vi "getServerCapability.vi"(8 "error in (no error)":errorcluster, 10 "ProtocolId in":string, 11 "IDeviceInfo in":refnum<class "IDeviceInfo.lvclass">) -> (0 "error out":errorcluster, 1 "ServerCapability out":refnum<class "IServerCapability.lvclass">, 2 "ProtocolId out":string, 3 "IDeviceInfo out":refnum<class "IDeviceInfo.lvclass">)   [LabVIEW 2022 SP3, in "openDAQ.lvlib" / "IBaseObject.lvlib" / "IPropertyObject.lvlib" / "IDeviceInfo.lvlib" / "IDeviceInfo.lvclass"]
uses:
  <instrlib>/openDAQ/Public/Classes/IDeviceInfo/IDeviceInfo.lvclass
  <instrlib>/openDAQ/Public/Classes/IDeviceInfo/IDeviceInfo.lvclass/IDeviceInfo.ctl
  <instrlib>/openDAQ/Public/Classes/daqCoreTypes/IString/IString.lvclass
  <instrlib>/openDAQ/Public/Classes/IServerCapability/IServerCapability.lvclass
  <instrlib>/openDAQ/Binaries/Windows/x86/copendaq32.dll
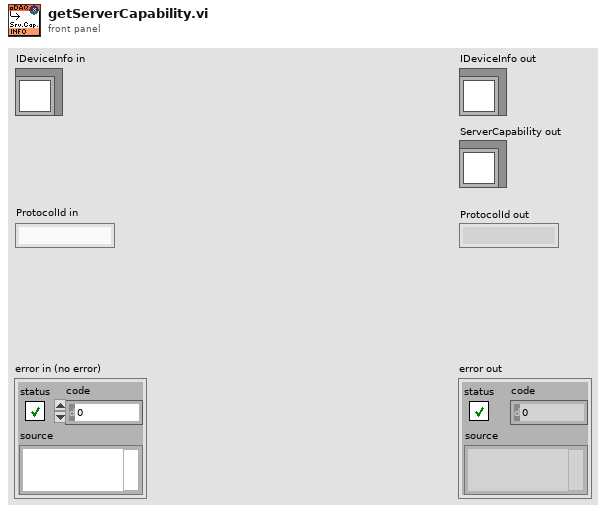
[diagram p1: front panel]
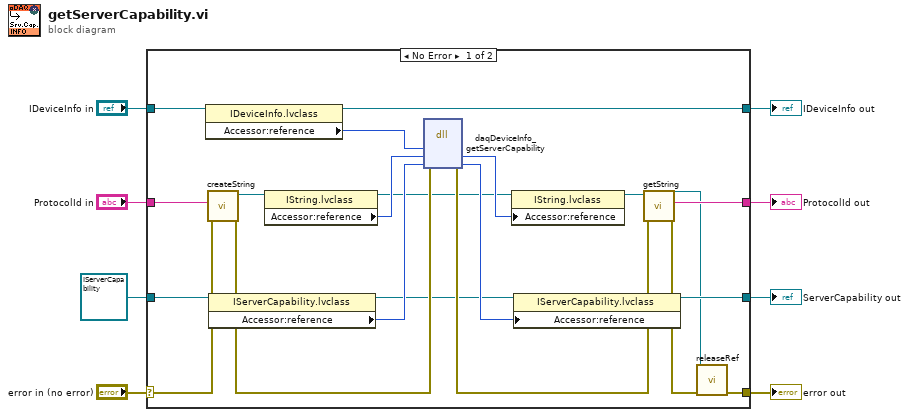
[diagram p0: block diagram]
diagram:
  n1 = case shown="No Error" "error in (no error)" {
    selector: "error in (no error)" -> [w17 w31]
    tunnel: [w11 w31] -> w7
    tunnel: [w22 w30] -> w5
    tunnel: "IDeviceInfo in" -> [w24 w30]
    tunnel: refnum<class "IServerCapability.lvclass"> refnum -> [w21 _]
    tunnel: [w20 _] -> w3
    tunnel: "ProtocolId in" -> [w19 _]
    tunnel: [w13 _] -> w1
    frame No Error {
      n2 = property class="IDeviceInfo.lvclass"(reference=w24) -> (reference out=w22:refnum<class "IDeviceInfo.lvclass">, "Accessor:reference"=w23:i64)  [unwired: 1 in, 1 out]
      n3 = call <instrlib>:"createString.vi"("error in (no error)"=w17, "String"=w19) -> ("error out"=w26:errorcluster, "IString out"=w18:refnum<class "IString.lvclass">)  [unwired: 8 in]
      n4 = property class="IServerCapability.lvclass"(reference=w21) -> (reference out=w25:refnum<class "IServerCapability.lvclass">, "Accessor:reference"=w29:i64)  [unwired: 1 in, 1 out]
      n5 = property class="IString.lvclass"(reference=w18) -> (reference out=w9:refnum<class "IString.lvclass">, "Accessor:reference"=w16:i64)  [unwired: 1 in, 1 out]
      n6 = dll-call lib="C:/Program Files (x86)/National Instruments/LabVIEW 2022/instr.lib/openDAQ/Binaries/Windows/x86/copendaq*.*" fn="daqDeviceInfo_getServerCapability"(error in=w26, "deviceInfo"=w23, "protocolId"=w16, "serverCapability"=w29) -> (error out=w27:errorcluster, "protocolId"=w15:i64, "serverCapability"=w28:i64)  [unwired: 4 in, 1 out]
      n7 = property class="IString.lvclass"(reference=w9, "Accessor:reference"=w15) -> (reference out=w14:refnum<class "IString.lvclass">)  [unwired: 1 in, 1 out]
      n8 = property class="IServerCapability.lvclass"(reference=w25, "Accessor:reference"=w28) -> (reference out=w20:refnum<class "IServerCapability.lvclass">)  [unwired: 1 in, 1 out]
      n9 = call <instrlib>:"getString.vi"("error in (no error)"=w27, "IString in"=w14) -> ("error out"=w12:errorcluster, "String out"=w13:string, "IString out"=w10:refnum<class "IString.lvclass">)  [unwired: 7 in]
      n10 = call-dynamic "releaseRef.vi"("error in (no error)"=w12, "IBaseObject in"=w10) -> ("error out"=w11:errorcluster)  [unwired: 9 in]
    }
    frame Error {
    }
  }
  "error out" <- w7
  "IDeviceInfo out" <- w5
  "ServerCapability out" <- w3
  "ProtocolId out" <- w1
